vi "RS485发送接收.vi"() -> ()   [LabVIEW 2010]
uses:
  <vilib>/Instr/_visa.llb/VISA Configure Serial Port (Instr).vi
panel:
  out "成功_2？ 2":bool caption="成功？"
  out "接收数据_2 2":string
  in  "发送数据_2":string
  in  "btn_关闭":bool
  in  "btn_开始测试":bool
  out "接收数据_1":string
  out "成功_1？":bool caption="成功？"
  in  "发送数据_1":string
  # "RS485测试界面"
  # "1#发送字符"
  # "2#发送字符"
  # "1#接收字符"
  # "2#接收字符"
  # "1#测试结果"
  # "2#测试结果"
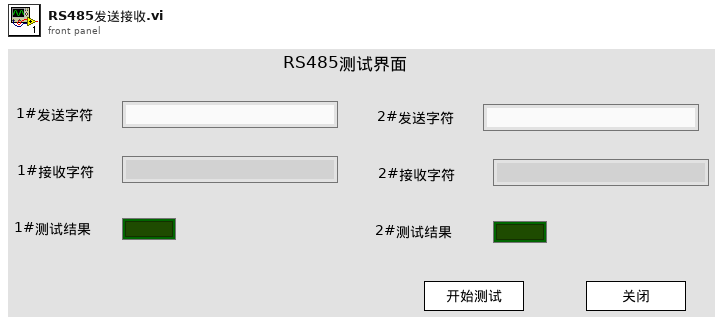
[diagram p1: front panel]
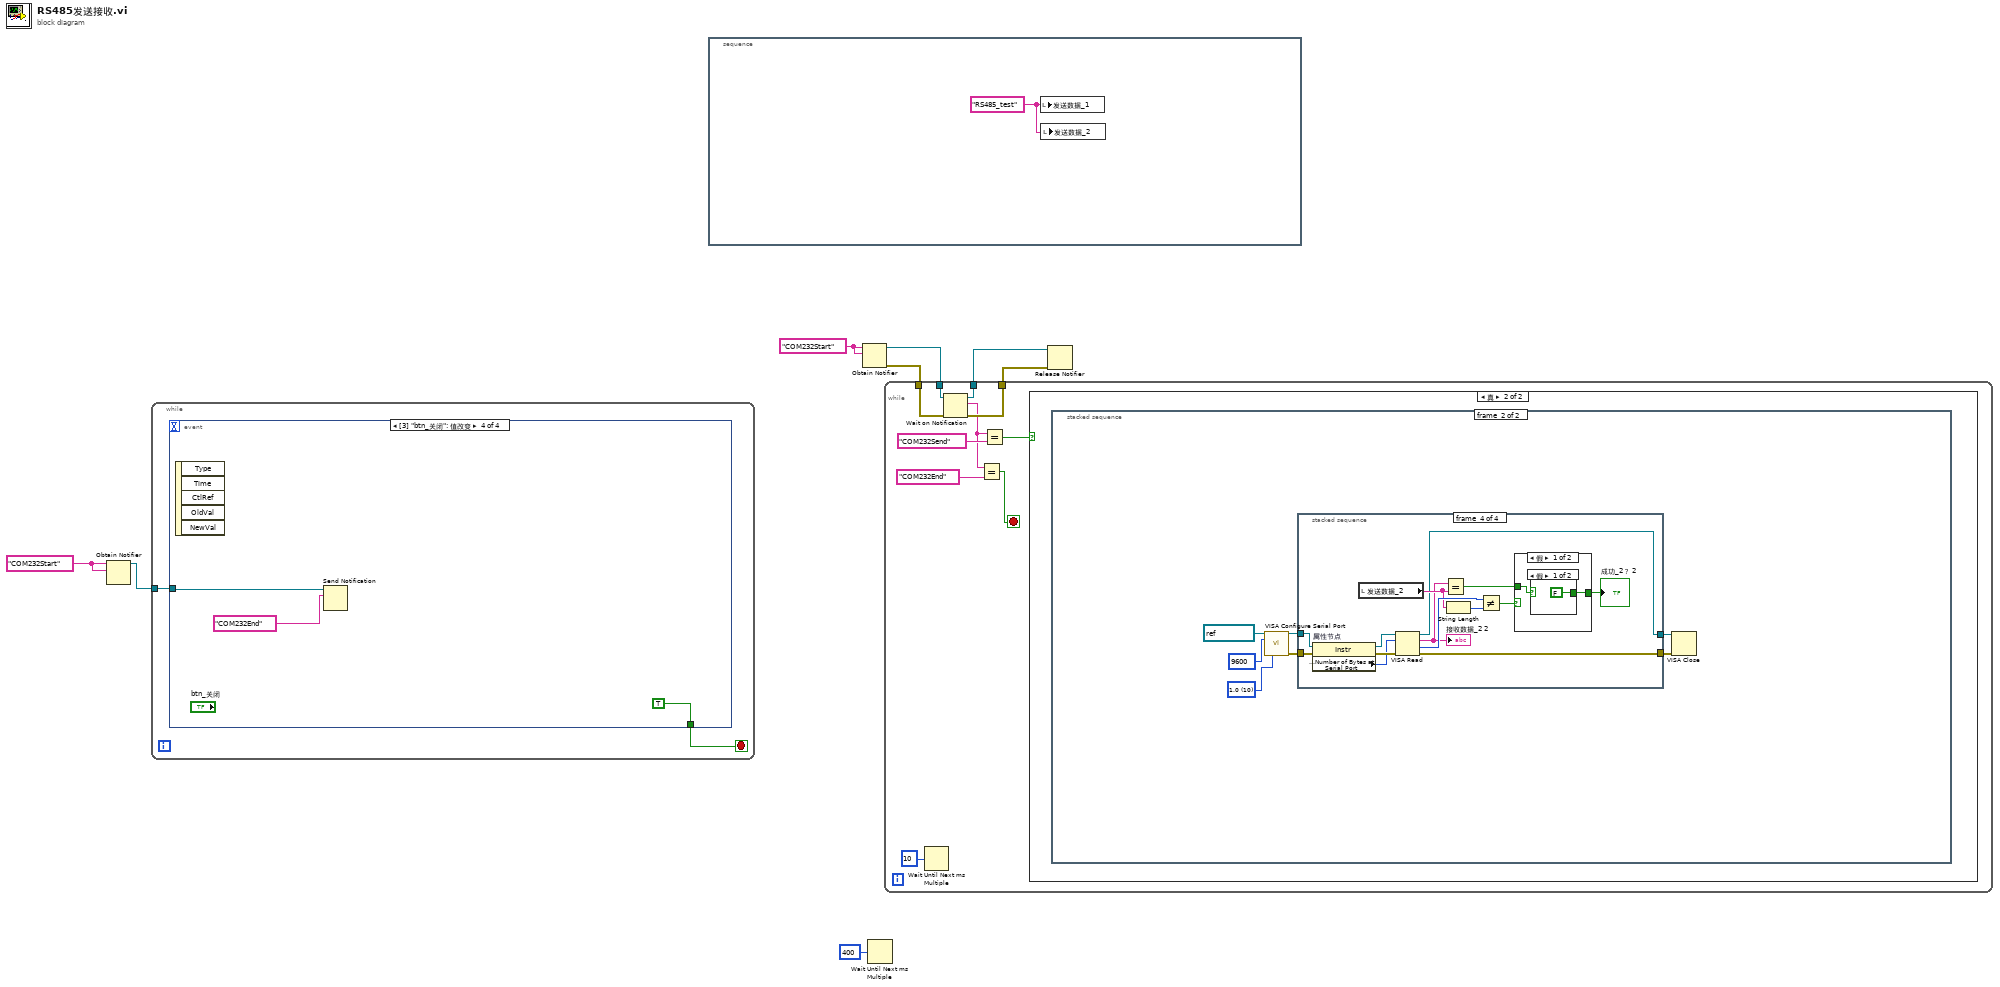
[diagram p0: block diagram]
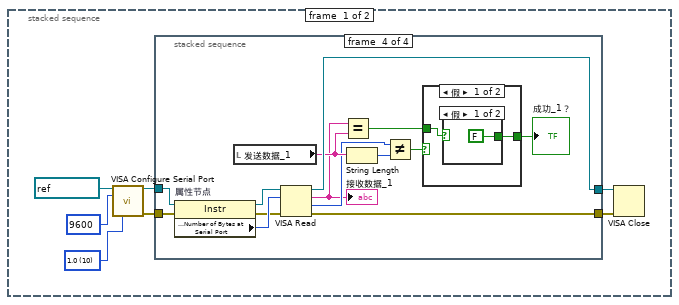
[diagram p3: hidden frame]
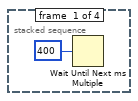
[diagram p4: hidden frame]
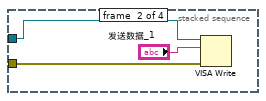
[diagram p5: hidden frame]
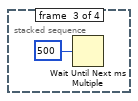
[diagram p6: hidden frame]
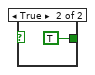
[diagram p7: hidden frame]
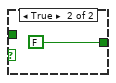
[diagram p8: hidden frame]
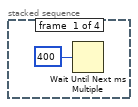
[diagram p9: hidden frame]
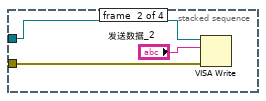
[diagram p10: hidden frame]
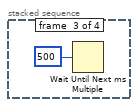
[diagram p11: hidden frame]
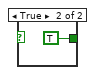
[diagram p12: hidden frame]
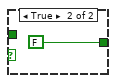
[diagram p13: hidden frame]
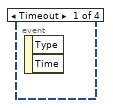
[diagram p14: hidden frame]
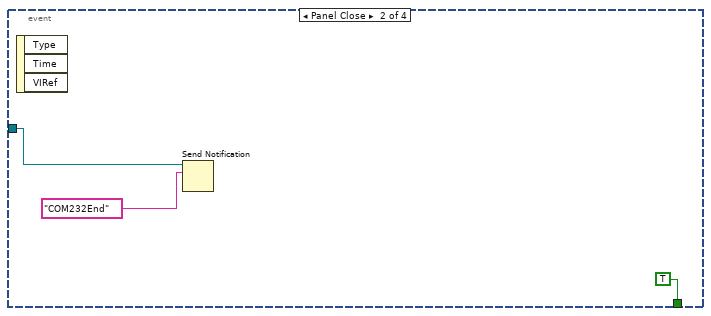
[diagram p15: hidden frame]
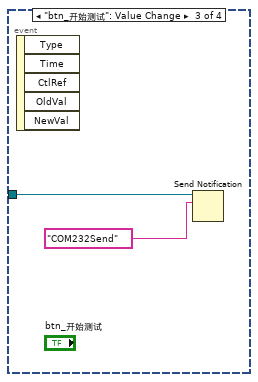
[diagram p16: hidden frame]
diagram:
  w3 = "COM232Start" ("名称（未命名）")
  w8 = "COM232Start" ("名称（未命名）")
  n1 = Obtain Notifier(name (unnamed)=w3, notification data type=w3) -> (notifier out=w2:refnum<notifier>)  [unwired: 2 in, 2 out]
  n2 = while {
    tunnel: w2 -> [w9]
    stop <- w10 stop-if-true
    n3 = event shown="[3] \"btn_关闭\": 值改变" {
      selector: _ -> [_ _ _ _]
      dyn-events: _ -> [_ _ _ _]
      timeout: _ -> [_ _ _ _]
      tunnel: [_ TRUE _ TRUE] -> w10
      tunnel: w9 -> [_ w11 w14 w16]
      event Timeout {
        n4 = event-data() -> ()  [unwired: 1 in, 2 out]
      }
      event Panel Close {
        n5 = event-data() -> ()  [unwired: 1 in, 3 out]
        n6 = Send Notification(notification="COM232End" ("通知"), notifier=w11) -> ()  [unwired: 1 in, 2 out]
      }
      event "btn_开始测试": Value Change {
        n7 = event-data() -> ()  [unwired: 1 in, 5 out]
        n8 = Send Notification(notification="COM232Send" ("通知"), notifier=w14) -> ()  [unwired: 1 in, 2 out]
      }
      event "btn_关闭": Value Change {
        n9 = event-data() -> ()  [unwired: 1 in, 5 out]
        n10 = Send Notification(notification="COM232End" ("通知"), notifier=w16) -> ()  [unwired: 1 in, 2 out]
      }
    }
  }
  n11 = stacked-sequence {
    frame #0 {
      w19 = "RS485_test" ("发送数据_1")
      n12 = local write "发送数据_1"(w19) -> ()
      n13 = local write "发送数据_2"(w19) -> ()
    }
  }
  n14 = Obtain Notifier(name (unnamed)=w8, notification data type=w8) -> (notifier out=w7:refnum<notifier>, error out=w6:errorcluster)  [unwired: 2 in, 1 out]
  n15 = Wait Until Next ms Multiple(millisecond multiple=u32 400 ("毫秒倍数")) -> ()  [unwired: 1 out]
  n16 = while {
    tunnel: w7 -> [w29]
    tunnel: w6 -> [w28]
    tunnel: [w27] -> w5
    tunnel: [w26] -> w4
    stop <- w21 stop-if-true
    n17 = Wait Until Next ms Multiple(millisecond multiple=u32 10 ("毫秒倍数")) -> ()  [unwired: 1 out]
    n18 = Wait on Notification(notifier=w29, error in (no error)=w28) -> (notifier out=w27:refnum<notifier>, notification=w23:string, error out=w26:errorcluster)  [unwired: 2 in, 1 out]
    n19 = Equal?(x=w23, y="COM232End" ("通知")) -> (x = y?=w21:bool)
    n20 = Equal?(x=w23, y="COM232Send" ("通知")) -> (x = y?=w24:bool)
    n21 = case shown="真" w24 {
      frame False {
      }
      frame True {
        n22 = stacked-sequence {
          frame #0 {
            w34 = u16 10 items=["1.0"=10, "1.5"=15, "2.0"=20] ("stop bits (10: 1 bit)")
            n23 = call-poly "VISA Configure Serial Port"("VISA resource name"=refnum<visa-resource-name> "COM4" ("R232端口"), "baud rate (9600)"=u32 9600, "stop bits (10: 1 bit)"=w34) -> ("VISA resource name out"=w33:refnum<visa-resource-name>, "error out"=w32:errorcluster)  [unwired: 11 in]
            n24 = stacked-sequence {
              tunnel: w33 -> [_ w40 _ w53]
              tunnel: w32 -> [_ w39 _ w52]
              tunnel: [_ _ _ w55] -> w30
              tunnel: [_ _ _ w54] -> w31
              frame #0 {
                n25 = Wait Until Next ms Multiple(millisecond multiple=u32 400 ("毫秒倍数")) -> ()  [unwired: 1 out]
              }
              frame #1 {
                n26 = VISA Write(VISA resource name=w40, write buffer="发送数据_1", error in (no error)=w39) -> ()  [unwired: 3 out]
              }
              frame #2 {
                n27 = Wait Until Next ms Multiple(millisecond multiple=u32 500 ("毫秒倍数")) -> ()  [unwired: 1 out]
              }
              frame #3 {
                n28 = property on="属性节点" class="Instr"(reference=w53, error in=w52) -> (reference out=w49:refnum<visa-resource-name>, error out=w47:errorcluster, "Serial Settings:Number of Bytes at Serial Port"=w48:u32)
                n29 = local read "发送数据_1"() -> (w46:string)
                n30 = VISA Read(VISA resource name=w49, byte count=w48, error in (no error)=w47) -> (VISA resource name out=w55:refnum<visa-resource-name>, read buffer=w42:string, return count=w45:u32, error out=w54:errorcluster)
                "接收数据_1" <- w42
                n31 = Equal?(x=w42, y=w46) -> (x = y?=w51:bool)
                n32 = String Length(string=w46) -> (length=w44:i32)
                n33 = Not Equal?(x=w45, y=w44) -> (x != y?=w43:bool)
                n34 = case shown="假" w43 {
                  tunnel: w51 -> [w57 _]
                  tunnel: [w56 FALSE] -> w50
                  frame False {
                    n35 = case shown="假" w57 {
                      tunnel: [FALSE TRUE] -> w56
                      frame False {
                      }
                      frame True {
                      }
                    }
                  }
                  frame True {
                  }
                }
                "成功_1？" <- w50
              }
            }
            n36 = VISA Close(VISA resource name=w30, error in (no error)=w31) -> ()  [unwired: 1 out]
          }
          frame #1 {
            w65 = u16 10 items=["1.0"=10, "1.5"=15, "2.0"=20] ("stop bits (10: 1 bit)")
            n37 = call-poly "VISA Configure Serial Port"("VISA resource name"=refnum<visa-resource-name> "COM5" ("R232端口"), "baud rate (9600)"=u32 9600, "stop bits (10: 1 bit)"=w65) -> ("VISA resource name out"=w62:refnum<visa-resource-name>, "error out"=w61:errorcluster)  [unwired: 11 in]
            n38 = stacked-sequence {
              tunnel: w62 -> [_ w71 _ w76]
              tunnel: w61 -> [_ w70 _ w75]
              tunnel: [_ _ _ w73] -> w66
              tunnel: [_ _ _ w74] -> w67
              frame #0 {
                n39 = Wait Until Next ms Multiple(millisecond multiple=u32 400 ("毫秒倍数")) -> ()  [unwired: 1 out]
              }
              frame #1 {
                n40 = VISA Write(VISA resource name=w71, write buffer="发送数据_2", error in (no error)=w70) -> ()  [unwired: 3 out]
              }
              frame #2 {
                n41 = Wait Until Next ms Multiple(millisecond multiple=u32 500 ("毫秒倍数")) -> ()  [unwired: 1 out]
              }
              frame #3 {
                n42 = property on="属性节点" class="Instr"(reference=w76, error in=w75) -> (reference out=w86:refnum<visa-resource-name>, error out=w85:errorcluster, "Serial Settings:Number of Bytes at Serial Port"=w84:u32)
                n43 = local read "发送数据_2"() -> (w80:string)
                n44 = VISA Read(VISA resource name=w86, byte count=w84, error in (no error)=w85) -> (VISA resource name out=w73:refnum<visa-resource-name>, read buffer=w77:string, return count=w82:u32, error out=w74:errorcluster)
                "接收数据_2 2" <- w77
                n45 = Equal?(x=w77, y=w80) -> (x = y?=w79:bool)
                n46 = String Length(string=w80) -> (length=w83:i32)
                n47 = Not Equal?(x=w82, y=w83) -> (x != y?=w81:bool)
                n48 = case shown="假" w81 {
                  tunnel: w79 -> [w88 _]
                  tunnel: [w87 FALSE] -> w78
                  frame False {
                    n49 = case shown="假" w88 {
                      tunnel: [FALSE TRUE] -> w87
                      frame False {
                      }
                      frame True {
                      }
                    }
                  }
                  frame True {
                  }
                }
                "成功_2？ 2" <- w78
              }
            }
            n50 = VISA Close(VISA resource name=w66, error in (no error)=w67) -> ()  [unwired: 1 out]
          }
        }
      }
    }
  }
  n51 = Release Notifier(notifier=w5, error in (no error)=w4) -> ()  [unwired: 1 in, 3 out]
